vi "Global 1 extract image.vi"() -> ()   [LabVIEW 2014]
panel:
  out "Original Image":T1(plugin-control)
  out "Image with Extract":T1(plugin-control)
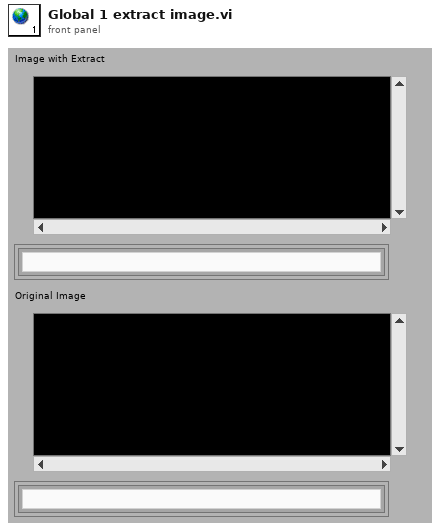
[diagram p1: front panel]
types:
  T1 = typedef "IMAQ Image.ctl" = refnum<image>
diagram:
